vi "Test App Get All Processes.vi"(8 "error in (no error)":errorcluster, 11 "Rig Test in":refnum<class "Application Dev Test.lvclass">) -> (0 "error out":errorcluster, 3 "Rig Test out":refnum<class "Application Dev Test.lvclass">)   [LabVIEW 2020, in "Application Dev Test.lvclass"]
uses:
  source/Framework Test Suite/Application Test/Application Test.lvclass/Application Test.ctl
  Application Dev Test.lvclass
  Application Dev Test.lvclass/Application Dev Test.ctl
  source/Framework/Process/Process.lvclass
  source/Framework/Application/Application.lvclass
  C:/Git/triarc-framework/source/Framework/Process/Process.lvclass
  C:/Git/triarc-framework/source/Framework/Base/Base.lvclass
  C:/Git/triarc-framework/source/Framework/Error Handler Interface/Error Handler Interface.lvclass
  C:/Git/triarc-framework/source/Framework/Logging/Logging.lvclass
  C:/Git/triarc-framework/source/Framework/Application/Application.lvclass
  C:/Git/triarc-framework/source/Framework/Async Handler/Async Handler.lvclass
  6f2e4378-1cf5-42ff-8d03-6273ee4332bb.vi
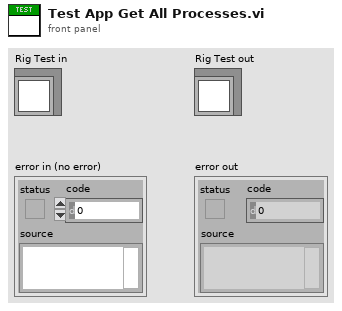
[diagram p1: front panel]
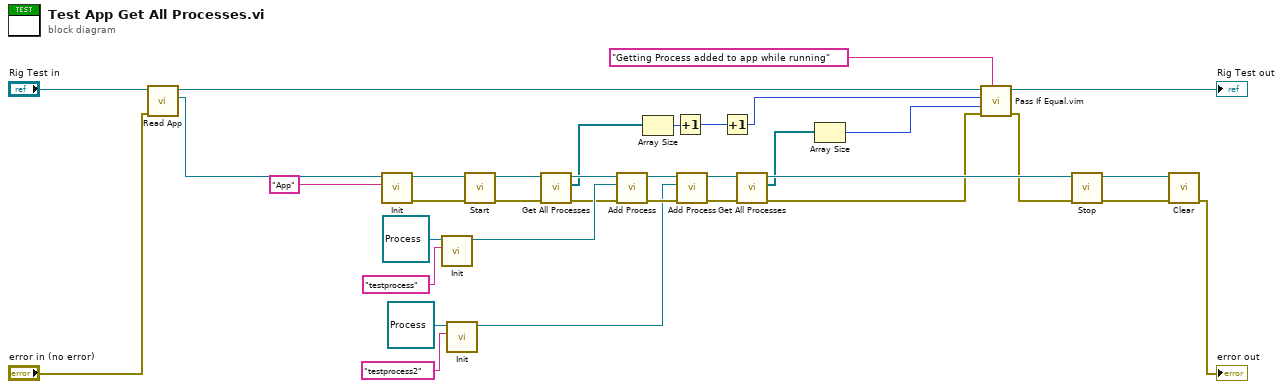
[diagram p0: block diagram]
diagram:
  n1 = call "Read App.vi"("error in (no error)"="error in (no error)", "Application Test In"="Rig Test in") -> ("App out"=w34:refnum<class "Application.lvclass">, "Application Test Out"=w22:refnum<class "Application Dev Test.lvclass">)  [unwired: 7 in, 1 out]
  n2 = call-dynamic "Init.vi"("Name"="App", "Process In"=w34) -> ("error out"=w23:errorcluster, "Process Out"=w24:refnum<class "Application.lvclass">)  [unwired: 8 in]
  n3 = call-dynamic "Init.vi"("Name"="testprocess", "Process In"=refnum<class "Process.lvclass"> refnum ("Process.lvclass")) -> ("Process Out"=w21:refnum<class "Process.lvclass">)  [unwired: 8 in, 1 out]
  n4 = call-dynamic "Init.vi"("Name"="testprocess2", "Process In"=refnum<class "Process.lvclass"> refnum ("Process.lvclass")) -> ("Process Out"=w8:refnum<class "Process.lvclass">)  [unwired: 8 in, 1 out]
  n5 = call "Start.vi"("error in (no error)"=w23, "Process In"=w24) -> ("error out"=w25:errorcluster, "Process Out"=w6:refnum<class "Application.lvclass">)  [unwired: 7 in, 1 out]
  n6 = call "Get All Processes.vi"("error in (no error)"=w25, "Application In"=w6) -> ("error out"=w7:errorcluster, "App Processes"=w1:refnum<class "Process.lvclass">[], "Application Out"=w5:refnum<class "Application.lvclass">)  [unwired: 7 in]
  n7 = call "Add Process.vi"("error in (no error)"=w7, "Process"=w21, "Application In"=w5) -> ("error out"=w29:errorcluster, "Application Out"=w15:refnum<class "Application.lvclass">)  [unwired: 7 in]
  n8 = Array Size(array=w1) -> (size(s)=w2:i32)
  n9 = Increment(x=w2) -> (x+1=w4:i32)
  n10 = call "Add Process.vi"("error in (no error)"=w29, "Process"=w8, "Application In"=w15) -> ("error out"=w16:errorcluster, "Application Out"=w14:refnum<class "Application.lvclass">)  [unwired: 7 in]
  n11 = Increment(x=w4) -> (x+1=w3:i32)
  n12 = call "Get All Processes.vi"("error in (no error)"=w16, "Application In"=w14) -> ("error out"=w12:errorcluster, "App Processes"=w11:refnum<class "Process.lvclass">[], "Application Out"=w32:refnum<class "Application.lvclass">)  [unwired: 7 in]
  n13 = Array Size(array=w11) -> (size(s)=w10:i32)
  n14 = call "Pass If Equal.vim"("Description"="Getting Process added to app while running", "error in (no error)"=w12, "Actual"=w10, "Expected"=w3, "LUnit Test Case In"=w22) -> ("error out"=w27:errorcluster, "LUnit Test Case Out"=→"Rig Test out":refnum<class "Application Dev Test.lvclass">)  [unwired: 5 in]
  n15 = call "Stop.vi"("error in (no error)"=w27, "Process In"=w32) -> ("error out"=w19:errorcluster, "Process Out"=w18:refnum<class "Application.lvclass">)  [unwired: 7 in, 1 out]
  n16 = call-dynamic "Clear.vi"("error in (no error)"=w19, "Application In"=w18) -> ("error out"=→"error out":errorcluster)  [unwired: 9 in]
